vi "AddAttribute.vi"(6 "Overwrite? (F)":bool, 8 "error in (no error)":errorcluster, 10 "Attribute":refnum<class "Attribute.lvclass">, 11 "SMO in":refnum<class "SMO.lvclass">) -> (0 "error out":errorcluster, 3 "SMO out":refnum<class "SMO.lvclass">)   [LabVIEW 2021, in "smo.lvlib" / "SMO.lvclass"]
uses:
  SMO.lvclass
  Support/Attribute/Attribute.lvclass
  SMO.lvclass/SMO.ctl
  Support/Attribute/Attribute.lvclass/Attribute.ctl
  <vilib>/Utility/LVClass/Get LV Class Name.vi
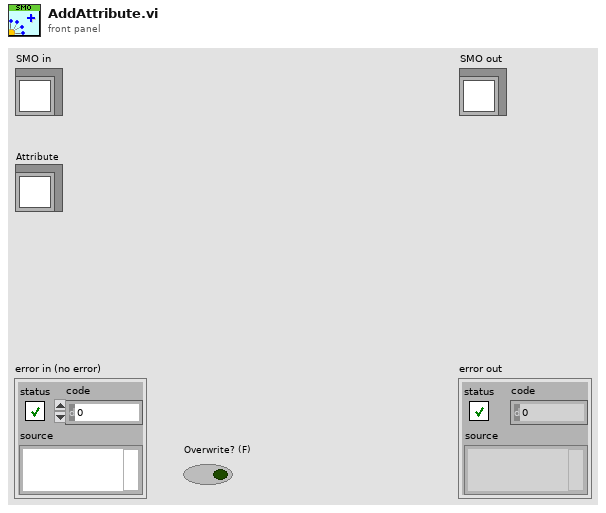
[diagram p1: front panel]
types:
  T1 = typedef "smo.lvlib/SMO.lvclass/PrivateData--Ref.ctl" = refnum<data-value>
  T2 = typedef "smo.lvlib/SMO.lvclass/PrivateData--Cluster.ctl" = cluster{"Parent Call":T3, "Registered Processes":T4[], "Sync Notifier":refnum<notifier>, "Process Error Notifier":refnum<notifier>, "Protected Events":T5, "Public Events":T6, "SMO State":T7, "[Attributes]":variant, "Launcher Close":refnum<notifier>, "Caller Watchdog":refnum<queue>, "Accessibility":T8, "NbStaticDependencies":u32}
  T3 = typedef "smo.lvlib/SMO.lvclass/Parent Call--Enum.ctl" = enum16{"Allows parent to run", "Does not request parent to run"}
  T4 = typedef "smo.lvlib/SMO.lvclass/RegisteredProcessData--Cluster.ctl" = cluster{"Name":string, "Static VI Ref":refnum<vi>, "Running":bool, "NotifierRef":u32}
  T5 = typedef "smo.lvlib/SMO.lvclass/Protected Events.ctl" = cluster{"StopProcesses":refnum<user-event>, "AbortProcesses":refnum<user-event>, "Config Changed":refnum<user-event>, "Dependency":refnum<user-event>}
  T6 = typedef "smo.lvlib/SMO.lvclass/Public Events.ctl" = cluster{"Error":refnum<user-event>, "State":refnum<user-event>, "Reserve State":refnum<user-event>}
  T7 = typedef "smo.lvlib/SMO.lvclass/SMOState --Enum.ctl" = enum16{"unknown", "Created", "Started", "Stopped"}
  T8 = typedef "smo.lvlib/SMO.lvclass/Accessibility--Cluster.ctl" = cluster{"Lock Key":string, "Reserve State":T9}
  T9 = typedef "smo.lvlib/SMO.lvclass/Reserve State--Enum.ctl" = enum16{"Unreserved", "Reserved", "Self-locked"}
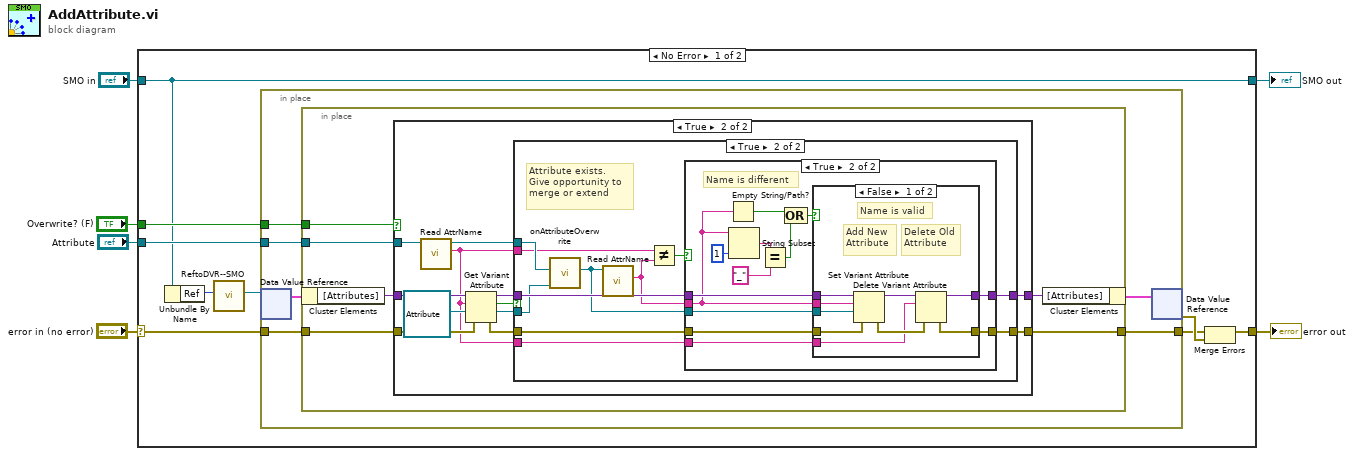
[diagram p0: block diagram]
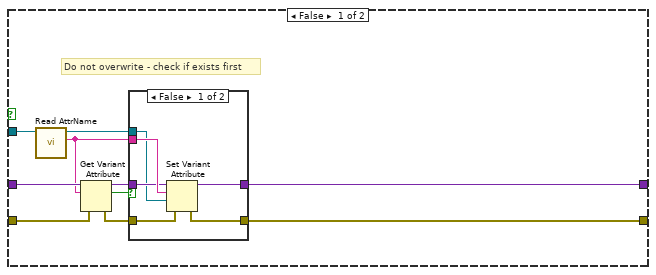
[diagram p2: hidden frame]
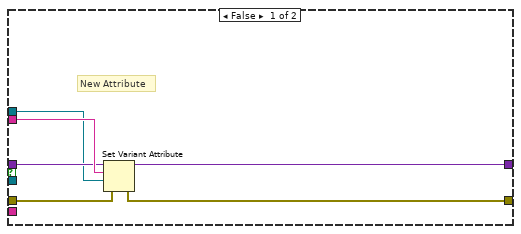
[diagram p4: hidden frame]
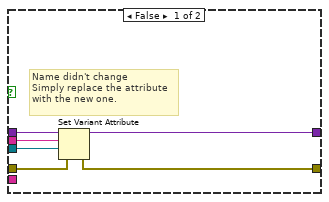
[diagram p5: hidden frame]
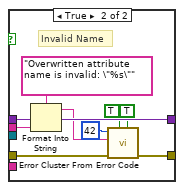
[diagram p6: hidden frame]
diagram:
  n1 = case shown="No Error" "error in (no error)" {
    selector: "error in (no error)" -> [w12 w113]
    tunnel: [w7 w112] -> w6
    tunnel: [w15 w113] -> w5
    tunnel: "Overwrite? (F)" -> [w14 _]
    tunnel: "Attribute" -> [w13 _]
    tunnel: "SMO in" -> [w7 w112]
    frame No Error {
      n2 = Unbundle By Name(w7) -> ("Ref"=w11:u32)
      n3 = call "ReftoDVR--SMO.vi"("Ref"=w11) -> ("Ref"=w10:T1)  [unwired: 10 in]
      n4 = in-place {
        in-place-border: w13 -> [w21]
        in-place-border: w14 -> [w18]
        in-place-border: w12 -> [w17]
        in-place-border: [w16] -> w8
        n5 = in-place-dvr #1(w10) -> (w20:T2)  [unwired: 1 out]
        n6 = in-place {
          in-place-border: w21 -> [w25]
          in-place-border: w18 -> [w24]
          in-place-border: w17 -> [w23]
          in-place-border: [w22] -> w16
          n7 = in-place-cluster #2(w20) -> ("[Attributes]"=w27:variant)
          n8 = case shown="True" w24 {
            tunnel: w27 -> [w37 w57]
            tunnel: [w36 w56] -> w26
            tunnel: w25 -> [w32 w49]
            tunnel: w23 -> [w28 w50]
            tunnel: [w35 w55] -> w22
            frame False {
              # "Do not overwrite - check if exists first"
              n9 = call "Read AttrName.vi"("Attribute in"=w32) -> ("Attribute Name"=w31:string, "Attribute out"=w30:refnum<class "Attribute.lvclass">)  [unwired: 8 in, 1 out]
              n10 = Get Variant Attribute(Variant=w37, name=w31, error in=w28) -> (duplicate Variant=w34:variant, found=w33:bool, error out=w29:errorcluster)  [unwired: 1 in, 1 out]
              n11 = case shown="False" w33 {
                tunnel: [w43 w45] -> w36
                tunnel: [w38 w44] -> w35
                tunnel: w31 -> [w42 _]
                tunnel: w34 -> [w41 w45]
                tunnel: w29 -> [w39 w44]
                tunnel: w30 -> [w40 _]
                frame False {
                  n12 = Set Variant Attribute(Variant=w41, name=w42, value=w40, error in=w39) -> (Variant out=w43:variant, error out=w38:errorcluster)  [unwired: 1 out]
                }
                frame True {
                }
              }
            }
            frame True {
              n13 = call "Read AttrName.vi"("Attribute in"=w49) -> ("Attribute Name"=w46:string, "Attribute out"=w52:refnum<class "Attribute.lvclass">)  [unwired: 8 in, 1 out]
              n14 = Get Variant Attribute(Variant=w57, name=w46, default value (empty Variant)=refnum<class "Attribute.lvclass"> refnum ("Attribute"), error in=w50) -> (duplicate Variant=w54:variant, found=w53:bool, value=w48:refnum<class "Attribute.lvclass">, error out=w51:errorcluster)
              n15 = case shown="True" w53 {
                tunnel: [w63 w74] -> w56
                tunnel: [w58 w71] -> w55
                tunnel: w46 -> [w62 w65]
                tunnel: w54 -> [w61 w73]
                tunnel: w51 -> [w59 w72]
                tunnel: w52 -> [w60 w70]
                tunnel: w48 -> [_ w69]
                tunnel: w46 -> [_ w64]
                frame False {
                  # "New Attribute"
                  n16 = Set Variant Attribute(Variant=w61, name=w62, value=w60, error in=w59) -> (Variant out=w63:variant, error out=w58:errorcluster)  [unwired: 1 out]
                }
                frame True {
                  # "Attribute exists.\nGive opportunity to\nmerge or extend"
                  n17 = call-dynamic "onAttributeOverwrite.vi"("Current Attribute"=w69, "New Attribute"=w70) -> ("Attribute out"=w68:refnum<class "Attribute.lvclass">)  [unwired: 9 in]
                  n18 = call "Read AttrName.vi"("Attribute in"=w68) -> ("Attribute Name"=w66:string)  [unwired: 8 in, 2 out]
                  n19 = Not Equal?(x=w65, y=w66) -> (x != y?=w67:bool)
                  n20 = case shown="True" w67 {
                    tunnel: [w80 w83] -> w74
                    tunnel: w73 -> [w79 w88]
                    tunnel: w72 -> [w78 w85]
                    tunnel: [w77 w84] -> w71
                    tunnel: w68 -> [w76 w86]
                    tunnel: w66 -> [w75 w82]
                    tunnel: w64 -> [_ w81]
                    frame False {
                      # "Name didn't change\nSimply replace the attribute\nwith the new one."
                      n21 = Set Variant Attribute(Variant=w79, name=w75, value=w76, error in=w78) -> (Variant out=w80:variant, error out=w77:errorcluster)  [unwired: 1 out]
                    }
                    frame True {
                      # "Name is different"
                      n22 = Empty String/Path?(string/path=w82) -> (empty?=w89:bool)
                      n23 = String Subset(string=w82, length (rest)=1 ("length (rest)")) -> (substring=w92:string)  [unwired: 1 in]
                      n24 = Equal?(x=w92, y="_") -> (x = y?=w90:bool)
                      n25 = Compound Arithmetic op=OR(w89, w90) -> (w87:bool)
                      n26 = case shown="False" w87 {
                        tunnel: w88 -> [w100 w111]
                        tunnel: w86 -> [w102 _]
                        tunnel: w82 -> [w101 w105]
                        tunnel: w85 -> [w99 w110]
                        tunnel: [w95 w109] -> w84
                        tunnel: [w97 w111] -> w83
                        tunnel: w81 -> [w94 _]
                        frame False {
                          # "Name is valid"
                          # "Delete Old\nAttribute"
                          # "Add New\nAttribute"
                          n27 = Set Variant Attribute(Variant=w100, name=w101, value=w102, error in=w99) -> (Variant out=w98:variant, error out=w96:errorcluster)  [unwired: 1 out]
                          n28 = Delete Variant Attribute(4:w96, 6:w94, 7:w98) -> (0:w95:errorcluster, 3:w97:variant)  [unwired: 1 out]
                        }
                        frame True {
                          # "Invalid Name"
                          n29 = Format Into String(format string="Overwritten attribute name is invalid: \"%s\"" ("error message (\"\")"), w105) -> (resulting string=w103:string)  [unwired: 2 in, 1 out]
                          n30 = call <vilib>:"Error Cluster From Error Code.vi"("is warning? (False)"=TRUE, "show call chain? (False)"=TRUE, "error in (no error)"=w110, "error message (\"\")"=w103, "error code (0)"=42 ("length (rest)")) -> ("error out"=w109:errorcluster)  [unwired: 4 in]
                        }
                      }
                    }
                  }
                }
              }
            }
          }
          n31 = in-place-cluster #2("[Attributes]"=w26) -> (w19:T2)
        }
        n32 = in-place-dvr #1(w19) -> (w9:errorcluster)  [unwired: 1 out]
      }
      n33 = Merge Errors(w8, w9) -> (w15:errorcluster)
    }
    frame Error {
    }
  }
  "error out" <- w5
  "SMO out" <- w6
